vi "Attack.vi"(11 "AI Manager in":refnum<class "AI Manager.lvclass">) -> (2 "Direction out":cluster{dbl, dbl}, 5 "Boost ?":bool)   [LabVIEW 2024, in "AI Manager.lvclass"]
doc: "MIT Licence\nCopyright (c) 2024 David Grollier"
uses:
  AI Manager.lvclass
  AI Manager.lvclass/AI Manager.ctl
  Game Componants/Game Componants.lvclass/Game Componants.ctl
  Game Componants/Game Board Component/Movable/Movable.lvclass/Movable.ctl
  Game Componants/Game Board Component/Movable/Flying Saucer/Flying Saucer.lvclass
  Game Componants/Game Board Component/Movable/Movable.lvclass
  Game Componants/Game Board/Game Board.lvclass
  Game Componants/Game Componants.lvclass
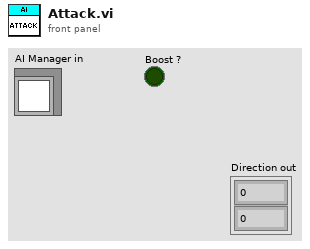
[diagram p1: front panel]
types:
  T1 = typedef "Velocity.ctl" = cluster{"Vx":dbl, "Vy":dbl}
  T2 = typedef "Coordinates.ctl" = cluster{"x":dbl, "y":dbl}
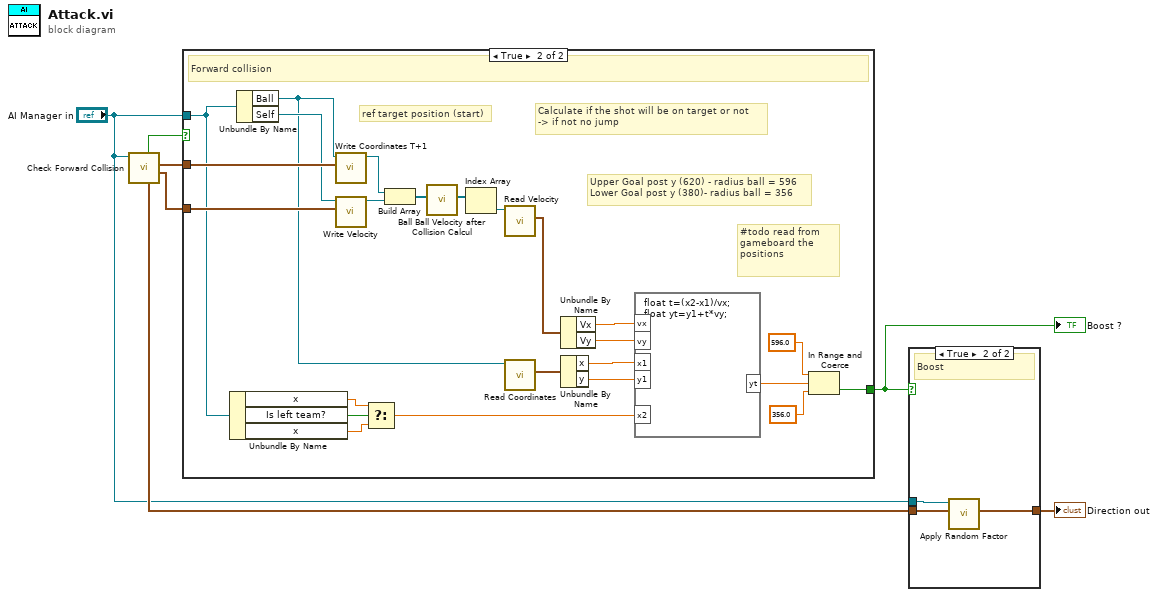
[diagram p0: block diagram]
diagram:
  n1 = call "Check Forward Collision.vi"("AI Manager in"="AI Manager in") -> ("Velocity out"=w6:T1, "Collision coordinate out"=w7:T1, "Vector direction out"=w4:cluster{dbl, dbl}, "Collision?"=w5:bool)  [unwired: 7 in]
  n2 = case shown="True" w5 {
    tunnel: w6 -> [_ w31]
    tunnel: w7 -> [_ w24]
    tunnel: "AI Manager in" -> [_ w21]
    tunnel: [_ w22] -> w2
    frame False {
      # "No forward collision"
    }
    frame True {
      # "Upper Goal post y (620) - radius ball = 596\nLower Goal post y (380)- radius ball = 356"
      # "#todo read from gameboard the positions"
      # "Calculate if the shot will be on target or not\n-> if not no jump"
      # "ref target position (start)"
      # "Forward collision"
      n3 = Unbundle By Name(w21) -> ("x"=w20:dbl, "Is left team?"=w19:bool, "x"=w18:dbl)
      n4 = Unbundle By Name(w21) -> ("Ball"=w17:refnum<class "Movable.lvclass">, "Self"=w23:refnum<class "Flying Saucer.lvclass">)
      n5 = call "Write Coordinates T+1.vi"("Coordinates"=w24, "Movable in"=w17) -> ("Movable out"=w27:refnum<class "Movable.lvclass">)  [unwired: 9 in]
      n6 = call "Write Velocity.vi"("Velocity"=w31, "Movable in"=w23) -> ("Movable out"=w28:refnum<class "Flying Saucer.lvclass">)  [unwired: 9 in]
      n7 = Select(t=w20, s=w19, f=w18) -> (s? t:f=w16:dbl)
      n8 = Build Array(w27, w28) -> (w29:refnum<class "Movable.lvclass">[])
      n9 = call "Ball Ball Velocity after Collision Calcul.vi"("Movables in"=w29) -> ("Movables out"=w30:refnum<class "Movable.lvclass">[])  [unwired: 10 in]
      n10 = Index Array(array=w30) -> (element=w26:refnum<class "Movable.lvclass">)  [unwired: 1 in]
      n11 = call-dynamic "Read Velocity.vi"("Movable in"=w26) -> ("Velocity"=w25:T1)  [unwired: 10 in]
      n12 = call "Read Coordinates.vi"("Game Componants in"=w17) -> ("Coordinates"=w15:T2)  [unwired: 10 in]
      n13 = Unbundle By Name(w25) -> ("Vx"=w14:dbl, "Vy"=w13:dbl)
      n14 = Unbundle By Name(w15) -> ("x"=w12:dbl, "y"=w11:dbl)
      n15 = formula code="float t=(x2-x1)/vx;\nfloat yt=y1+t*vy;"("x1"=w12, "x2"=w16, "vx"=w14, "y1"=w11, "vy"=w13) -> ("yt"=w10:dbl)
      n16 = In Range and Coerce(upper limit=596.0 ("y"), x=w10, lower limit=356.0 ("y")) -> (In Range?=w22:bool)  [unwired: 1 out]
    }
  }
  "Boost ?" <- w2
  n17 = case shown="True" w2 {
    tunnel: w4 -> [w32 w35]
    tunnel: "AI Manager in" -> [_ w34]
    tunnel: [w32 w33] -> w1
    frame False {
      # "No boost"
    }
    frame True {
      # "Boost"
      n18 = call "Apply Random Factor.vi"("Velocity in"=w35, "AI Manager in"=w34) -> ("Adjusted Velocity out"=w33:cluster{dbl, dbl})  [unwired: 9 in]
    }
  }
  "Direction out" <- w1
